vi "sv_Shift and Low Pass Filter (1 Channel) with IC.vi"(0 "input signal":dbl[](array[numeric]), 1 "reset? (F)":bool, 5 "t0":dbl, 7 "center":dbl, 9 "decimation factor":i32, 11 "error in (no error)":errorcluster, 12 "initial conditions":T1 {"filter settings"."filters"."coefficients" format="%.2f"}, 13 "new dt":dbl) -> (4 "enveloped signal":dbl[](array[numeric]), 6 "t0 out":dbl, 14 "final conditions":T1 {"filter settings"."filters"."coefficients" format="%.2f"}, 15 "error out":errorcluster)   [LabVIEW 2017, in "SoundVib_FaultAnalysis.lvlib"]
uses:
  <vilib>/addons/Sound and Vibration/Order Analysis/Fault Analysis/SoundVib_FaultAnalysis.lvlib
  <vilib>/addons/_NISVFA/_Shared subVIs/Controls/svc_Envelope Detection State.ctl
  <vilib>/addons/_NISVFA/_Shared subVIs/Controls/OAT Decimation Filter.ctl
  <vilib>/addons/Sound and Vibration/Order Analysis/Resample Order Tracking/SubVIs/OAT Frequency Shift (Mixer).vi
  <vilib>/addons/Sound and Vibration/Order Analysis/Resample Order Tracking/SubVIs/oa_Decimation with CIC and Compensation Filter.vi
  <vilib>/addons/Sound and Vibration/Order Analysis/Fault Analysis/SubVIs/oa_Demodulation Initial States (1 Channel).vi
  <vilib>/addons/Sound and Vibration/Order Analysis/Adv Resampling/OAT Single Stage Decimation with IC.vi
  <vilib>/addons/Sound and Vibration/Order Analysis/Resample Order Tracking/SubVIs/OAT CIC Decimation.vi
  <vilib>/addons/Sound and Vibration/Order Analysis/Resample Order Tracking/SubVIs/oa_Interpolate Zeros Between Samples.vi
  <vilib>/addons/Sound and Vibration/Order Analysis/Resample Order Tracking/SubVIs/oa_Calculate Delay of CIC Decimation Interpolation Filter.vi
  <vilib>/addons/Sound and Vibration/Order Analysis/Resample Order Tracking/SubVIs/oa_Create CIC Compensation Filter.vi
  <vilib>/addons/Sound and Vibration/Order Analysis/Resample Order Tracking/SubVIs/oa_Create CIC LP Truncation Filter.vi
  <vilib>/addons/Sound and Vibration/Order Analysis/Resample Order Tracking/SoundVib_Resampling.lvlib
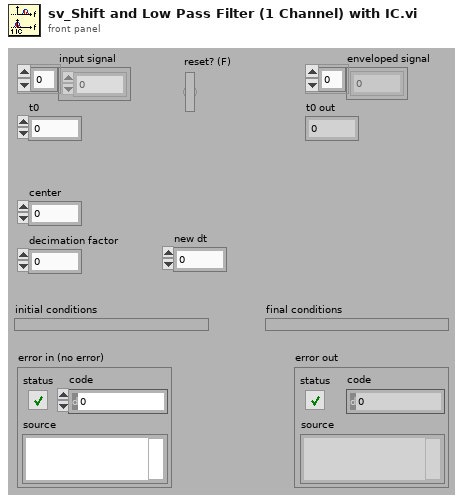
[diagram p1: front panel]
types:
  T1 = typedef "svc_Envelope Detection State.ctl" = cluster{"filter settings":cluster{"CIC Settings":cluster{"Numeric":i32, i32, i32}, "filters":T2[], "delay":i32, "interpolation factor":i32}, "filter state":cluster{"t0":dbl, "phase":dbl, "real filter state":cluster{cluster{dbl[]}, cluster{dbl[]}[]}, "imaginary filter state":cluster{cluster{dbl[]}, cluster{dbl[]}[]}, "delay":i32}, "reset pending":bool}
  T2 = typedef "OAT Decimation Filter.ctl" = cluster{"coefficients":dbl[], "factor":i32}
  T3 = cluster{"t0":dbl, "phase":dbl, "real filter state":cluster{cluster{dbl[]}, cluster{dbl[]}[]}, "imaginary filter state":cluster{cluster{dbl[]}, cluster{dbl[]}[]}, "delay":i32}
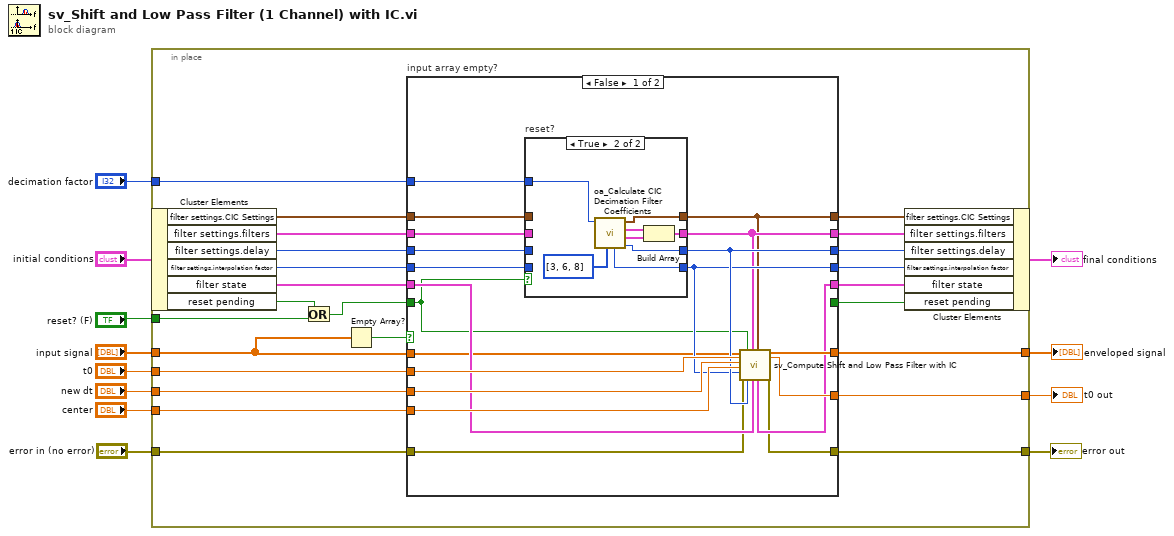
[diagram p0: block diagram]
diagram:
  n1 = in-place {
    in-place-border: "input signal" -> [w15]
    in-place-border: "decimation factor" -> [w36]
    in-place-border: "center" -> [w35]
    in-place-border: "t0" -> [w34]
    in-place-border: [w33] -> w8
    in-place-border: "new dt" -> [w32]
    in-place-border: "reset? (F)" -> [w19]
    in-place-border: [w31] -> w5
    in-place-border: "error in (no error)" -> [w14]
    in-place-border: [w13] -> w1
    n2 = in-place-cluster #1("initial conditions") -> ("filter settings.CIC Settings"=w28:cluster{"Numeric":i32, i32, i32}, "filter settings.filters"=w27:T2[], "filter settings.delay"=w26:i32, "filter settings.interpolation factor"=w25:i32, "filter state"=w30:T3, "reset pending"=w20:bool)
    n3 = Or(x=w20, y=w19) -> (x .or. y?=w18:bool)
    n4 = Empty Array?(array=w15) -> (empty?=w17:bool)
    n5 = case "input array empty?" shown="False" w17 {
      tunnel: w36 -> [w56 _]
      tunnel: w35 -> [w55 _]
      tunnel: w34 -> [w54 w70]
      tunnel: [w53 w70] -> w33
      tunnel: w32 -> [w52 _]
      tunnel: [w51 w71] -> w31
      tunnel: w30 -> [w50 w72]
      tunnel: [w49 w72] -> w29
      tunnel: w28 -> [w48 w76]
      tunnel: w27 -> [w47 w75]
      tunnel: w26 -> [w46 w74]
      tunnel: w25 -> [w45 w73]
      tunnel: [w37 w76] -> w24
      tunnel: [w38 w75] -> w23
      tunnel: [w44 w74] -> w22
      tunnel: [w43 w73] -> w21
      tunnel: w18 -> [w42 w77]
      tunnel: [_ w77] -> w16
      tunnel: w15 -> [w41 w71]
      tunnel: w14 -> [w40 w69]
      tunnel: [w39 w69] -> w13
      frame False {
        n6 = case "reset?" shown="True" w42 {
          tunnel: [w60 w68] -> w37
          tunnel: [w59 w65] -> w38
          tunnel: [w57 w64] -> w43
          tunnel: [w58 w63] -> w44
          tunnel: w56 -> [_ w62]
          tunnel: w48 -> [w60 _]
          tunnel: w47 -> [w59 _]
          tunnel: w46 -> [w58 _]
          tunnel: w45 -> [w57 _]
          frame False {
          }
          frame True {
            n7 = call <vilib>:"oa_Calculate CIC Decimation Filter Coefficients.vi"("CIC stages"=i32[] [3, 6, 8], "decimation/interpolation factor"=w62) -> ("delay"=w63:i32, "lp filter settings"=w66:T2, "compensation filter settings"=w67:T2, "CIC Settings"=w68:cluster{"Numeric":i32, i32, i32}, "interpolation factor"=w64:i32)  [unwired: 5 in]
            n8 = Build Array(w67, w66) -> (w65:T2[])
          }
        }
        n9 = call <vilib>:"sv_Compute Shift and Low Pass Filter with IC.vi"("input signal"=w41, "t0"=w54, "new dt"=w52, "center"=w55, "interpolation factor"=w43, "error in (no error)"=w40, "reset? (F)"=w42, "delay"=w44, "filters"=w38, "initial conditions"=w50, "CIC settings"=w37) -> ("final conditions"=w49:T3, "enveloped signal"=w51:dbl[], "t0 out"=w53:dbl, "error out"=w39:errorcluster)  [unwired: 5 in]
      }
      frame True {
      }
    }
    n10 = in-place-cluster #1("filter settings.CIC Settings"=w24, "filter settings.filters"=w23, "filter settings.delay"=w22, "filter settings.interpolation factor"=w21, "filter state"=w29, "reset pending"=w16) -> (→"final conditions":T1)
  }
  "enveloped signal" <- w5
  "t0 out" <- w8
  "error out" <- w1
